vi "Open-characteristic-file-references.vi"(8 "error in":errorcluster, 11 "Storage params. ref. in":refnum<data-value>) -> (0 "error IO":errorcluster, 3 "Storage params. ref.":refnum<data-value>)   [LabVIEW 2013, in "CameraVision.lvlib" / "CV-Storage.lvclass"]
doc: "This function opens access references to the characteristics file. In this file information about the image timing, image characteristics, melt-pool characteristics and temperature data is stored, when applicable. The file format is .tdms, which is a National Instruments proprietary binary format. It is compatible with Microsoft Excel, by using a free plugin.\n\nThe file path and name are the user specified 'Storage directory' and 'Base file name', appended with '-Characteristics'. Any existing file with the same name is erased.\n\nIf \"one file for each layer\" is selected in the 'Storage' options, a new file will be created for each layer/iteration. If a file with the same name and iteration number exists, it will be overwritten.\nIf \"one file for all layers\" is selected, a new file is only created for the first layer/iteration. Subsequent iterations will append to the first file."
uses:
  CV-Storage.lvclass
  CV-Storage.lvclass/CV-Storage.ctl
  Read Storage directory.vi
  Read Storage prefix.vi
  Read Storage labels.vi
  Write Characteristics file reference RW.vi
  Write Characteristics file reference RO.vi
  Write Temperature file reference W.vi
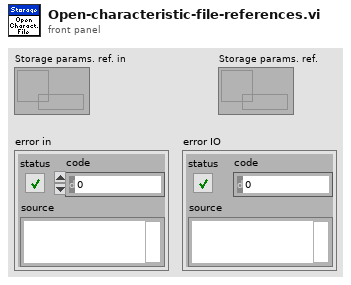
[diagram p1: front panel]
types:
  T1 = enum16{"open", "open or create", "create or replace", "create", "open (read-only)"}
  T2 = typedef "Storage-types-labels.ctl" = cluster{"Original":string, "Corrected":string, "Binary":string, "Temperature":string, "Characteristics":string, "Mapping":string, "TemperatureValues":string}
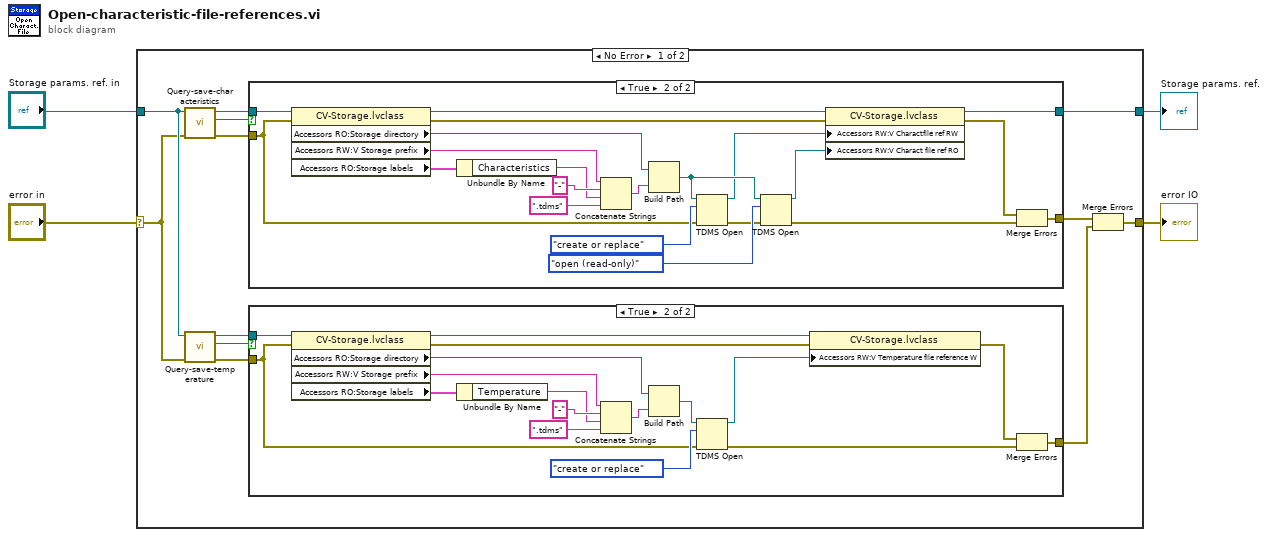
[diagram p0: block diagram]
diagram:
  n1 = case shown="No Error" "error in" {
    selector: "error in" -> [w10 w59]
    tunnel: [w6 w59] -> w4
    tunnel: "Storage params. ref. in" -> [w11 w58]
    tunnel: [w15 w58] -> w1
    frame No Error {
      n2 = call "Query-save-characteristics.vi"("error in"=w10, "Storage params. ref. in"=w11) -> ("error IO"=w13:errorcluster, "Save characteristics?"=w14:bool, "Storage params. ref."=w12:refnum<data-value>)  [unwired: 7 in]
      n3 = call "Query-save-temperature.vi"("error in"=w10, "Storage params. ref. in"=w11) -> ("error IO"=w7:errorcluster, "Save temperature?"=w9:bool, "Storage params. ref."=w8:refnum<data-value>)  [unwired: 7 in]
      n4 = case shown="True" w14 {
        tunnel: w12 -> [w36 w53]
        tunnel: [w35 w50] -> w16
        tunnel: [w36 w42] -> w15
        tunnel: w13 -> [w35 w41]
        frame False {
        }
        frame True {
          n5 = property class="CV-Storage.lvclass"(reference=w53, error in=w41) -> (reference out=w46:refnum<data-value>, error out=w49:errorcluster, "Accessors RO:Storage directory"=w52:path, "Accessors RW:V Storage prefix"=w51:string, "Accessors RO:Storage labels"=w38:T2)
          n6 = Unbundle By Name(w38) -> ("Characteristics"=w37:string)
          n7 = Concatenate Strings(w51, "-", w37, ".tdms" ("string")) -> (w47:string)
          n8 = Build Path(base path=w52, name or relative path=w47) -> (appended path=w57:path)
          n9 = TDMS Open(8:w41, 10:T1."create or replace" ("operation (0:open)"), 11:w57) -> (0:w55:errorcluster, 3:w44:refnum<k34>)  [unwired: 4 in]
          n10 = TDMS Open(8:w55, 10:T1."open (read-only)" ("operation (0:open)"), 11:w57) -> (0:w54:errorcluster, 3:w45:refnum<k34>)  [unwired: 4 in]
          n11 = property class="CV-Storage.lvclass"(reference=w46, error in=w49, "Accessors RW:V Charactfile ref RW"=w44, "Accessors RW:V Charact file ref RO"=w45) -> (reference out=w42:refnum<data-value>, error out=w48:errorcluster)
          n12 = Merge Errors(w48, w54) -> (w50:errorcluster)
        }
      }
      n13 = case shown="True" w9 {
        tunnel: w8 -> [_ w33]
        tunnel: [w17 w30] -> w5
        tunnel: w7 -> [w17 w23]
        frame False {
        }
        frame True {
          n14 = property class="CV-Storage.lvclass"(reference=w33, error in=w23) -> (reference out=w26:refnum<data-value>, error out=w29:errorcluster, "Accessors RO:Storage directory"=w32:path, "Accessors RW:V Storage prefix"=w31:string, "Accessors RO:Storage labels"=w20:T2)
          n15 = Unbundle By Name(w20) -> ("Temperature"=w19:string)
          n16 = Concatenate Strings(w31, "-", w19, ".tdms" ("string")) -> (w27:string)
          n17 = Build Path(base path=w32, name or relative path=w27) -> (appended path=w34:path)
          n18 = TDMS Open(8:w23, 10:T1."create or replace" ("operation (0:open)"), 11:w34) -> (0:w18:errorcluster, 3:w25:refnum<k34>)  [unwired: 4 in]
          n19 = property class="CV-Storage.lvclass"(reference=w26, error in=w29, "Accessors RW:V Temperature file reference W"=w25) -> (error out=w28:errorcluster)  [unwired: 1 out]
          n20 = Merge Errors(w28, w18) -> (w30:errorcluster)
        }
      }
      n21 = Merge Errors(w16, w5) -> (w6:errorcluster)
    }
    frame Error {
    }
  }
  "error IO" <- w4
  "Storage params. ref." <- w1
